vi "PH_Stepmotor_BaseClass.Data to Axis Information.vi"(0 "data":i8[](array[numeric]), 1 "Type Descriptor":string) -> (2 "Axis Information":T1)   [LabVIEW 2014, in "PH_Stepmotor_BaseClass.lvlib"]
uses:
  PH_Stepmotor_BaseClass.lvlib
  PH_Stepmotor_BaseClass.Axis Information.ctl
  PH_Stepmotor_BaseClass.Axis Activity.ctl
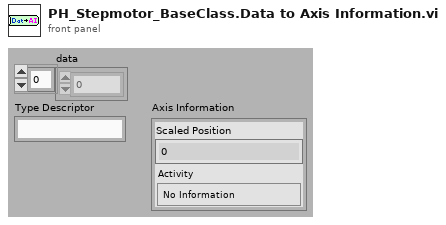
[diagram p1: front panel]
types:
  T1 = typedef "PH_Stepmotor_BaseClass.lvlib/PH_Stepmotor_BaseClass.Axis Information.ctl" = cluster{"Scaled Position":dbl, "Activity":T2}
  T2 = typedef "PH_Stepmotor_BaseClass.lvlib/PH_Stepmotor_BaseClass.Axis Activity.ctl" = enum16{"No Information", "stopped", "running", "Failure", "Alarm", "stopped at backward ES", "stopped at foreward ES"}
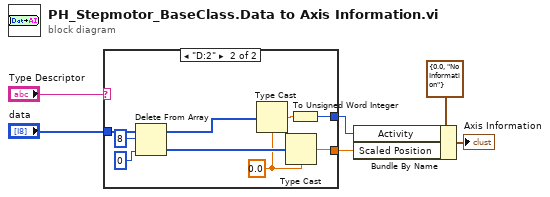
[diagram p0: block diagram]
diagram:
  n1 = case "Check data type" shown="\"D:2\"" "Type Descriptor" {
    tunnel: "data" -> [_ w15]
    tunnel: [_ w14] -> w2
    tunnel: [_ w9] -> w1
    frame Default {
    }
    frame "D:2" {
      w8 = 0.0
      n2 = Delete From Array(array=w15, length=8, index=0) -> (deleted portion=w13:i8[], array with subset deleted=w7:i8[])
      n3 = Type Cast(type=w8, x=w7) -> (*(type *) &x=w10:dbl)
      n4 = Type Cast(type=w8, x=w13) -> (*(type *) &x=w14:dbl)
      n5 = To Unsigned Word Integer(number=w10) -> (unsigned 16bit integer=w9:u16)
    }
  }
  n6 = Bundle By Name(cluster=T1 {"Scaled Position"=0.0, "Activity"=enum."No Information"} ("Axis Information"), "Activity"=w1, "Scaled Position"=w2) -> (→"Axis Information":T1)
